vi "Left Join.vi"(9 "Array 2":string[][](array[string]), 11 "Array 1":string[][](array[string])) -> (2 "Left Joined Array":string[][](array[string]))   [LabVIEW 2020]
uses:
  a75eeadb-a20a-426b-b48b-c9c06ab4b909.vi
  965599a9-35c5-4084-8906-0a043779e57e.vi
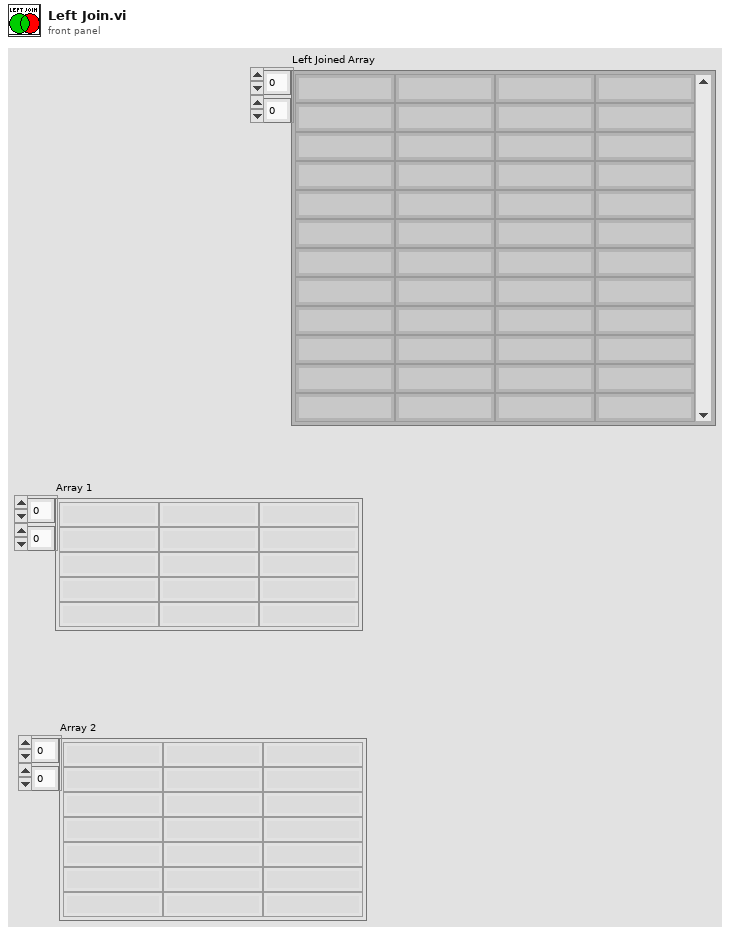
[diagram p1: front panel]
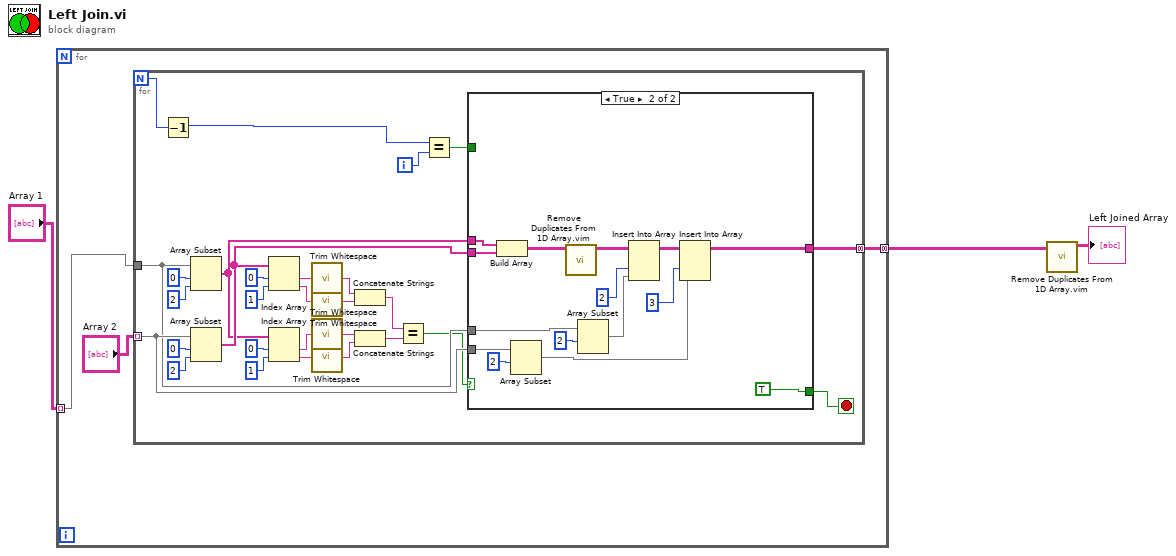
[diagram p0: block diagram]
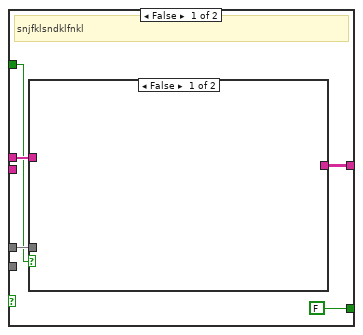
[diagram p2: hidden frame]
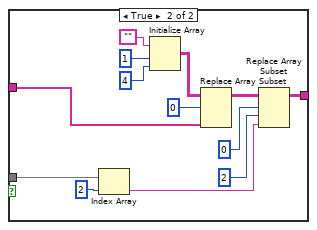
[diagram p3: hidden frame]
diagram:
  n1 = for {
    tunnel: "Array 1" -> [w5] mode=indexing
    tunnel: [w6] -> w2 mode=concatenating
    n2 = for {
      N -> [w26]
      tunnel: "Array 2" -> [w30] mode=indexing
      tunnel: w5 -> [w24]
      tunnel: [w35] -> w6 mode=concatenating
      i -> [w28]
      stop <- w29 stop-if-true
      n3 = Decrement(x=w26) -> (x-1=w25:i32)
      n4 = Array Subset(array=w24, index=0, length=2) -> (w22:string[])
      n5 = Array Subset(array=w30, index=0, length=2) -> (w23:string[])
      n6 = Index Array(array=w23, index #1=0 ("index"), index #2=1 ("index")) -> (element #1=w17:string, element #2=w16:string)
      n7 = Index Array(array=w22, index #1=0 ("index"), index #2=1 ("index")) -> (element #1=w15:string, element #2=w14:string)
      n8 = call <vilib>:"Trim Whitespace.vi"("string"=w17) -> ("trimmed string"=w11:string)  [unwired: 1 in]
      n9 = call <vilib>:"Trim Whitespace.vi"("string"=w16) -> ("trimmed string"=w10:string)  [unwired: 1 in]
      n10 = call <vilib>:"Trim Whitespace.vi"("string"=w15) -> ("trimmed string"=w12:string)  [unwired: 1 in]
      n11 = call <vilib>:"Trim Whitespace.vi"("string"=w14) -> ("trimmed string"=w13:string)  [unwired: 1 in]
      n12 = Concatenate Strings(w11, w10) -> (w9:string)
      n13 = Concatenate Strings(w12, w13) -> (w8:string)
      n14 = Equal?(x=w9, y=w8) -> (x = y?=w7:bool)
      n15 = Equal?(x=w25, y=w28) -> (x = y?=w27:bool)
      n16 = case shown="True" w7 {
        tunnel: [w38 w57] -> w35
        tunnel: w24 -> [w40 w64]
        tunnel: w30 -> [_ w61]
        tunnel: w22 -> [w39 w68]
        tunnel: w23 -> [_ w67]
        tunnel: [FALSE TRUE] -> w29
        tunnel: w27 -> [w36 _]
        frame False {
          # "snjfklsndklfnkl"
          n17 = case shown="False" w36 {
            tunnel: w40 -> [_ w52]
            tunnel: w39 -> [_ w44]
            tunnel: [_ w41] -> w38
            frame False {
            }
            frame True {
              n18 = Index Array(array=w52, index=2) -> (element=w49:string)
              n19 = Initialize Array("", 1 ("dimension size"), 4 ("dimension size")) -> (w45:string[][])
              n20 = Replace Array Subset(array=w45, new element=w44, index (row)=0) -> (w42:string[][])  [unwired: 1 in]
              n21 = Replace Array Subset(array=w42, new element=w49, index (row)=0 ("disabled index (row)"), index (col)=2 ("index (row)")) -> (w41:string[][])
            }
          }
        }
        frame True {
          n22 = Build Array(w68, w67) -> (w66:string[][])
          n23 = Array Subset(array=w61, index=2) -> (w58:string[])  [unwired: 1 in]
          n24 = call "Remove Duplicates From 1D Array.vim"("array"=w66) -> ("array with duplicates removed"=w65:string[][])  [unwired: 10 in]
          n25 = Array Subset(array=w64, index=2) -> (w63:string[])  [unwired: 1 in]
          n26 = Insert Into Array(array=w65, index (col)=2 ("index (row)"), new element=w63) -> (w59:string[][])  [unwired: 1 in]
          n27 = Insert Into Array(array=w59, index (col)=3 ("index (row)"), new element=w58) -> (w57:string[][])  [unwired: 1 in]
        }
      }
    }
  }
  n28 = call "Remove Duplicates From 1D Array.vim"("array"=w2) -> ("array with duplicates removed"=→"Left Joined Array":string[][])  [unwired: 10 in]
